vi "Configure Measure Mode.vi"(0 "VISA resource name":refnum<visa-resource-name>, 1 "MeasureMode (0=MyMeasure)":T1(ring), 5 "Show Table? (True)":bool=TRUE, 7 "Show Statistics? (True)":bool=TRUE, 9 "Show Histicons? (False)":bool, 11 "error in (no error)":errorcluster) -> (4 "VISA resource name out":refnum<visa-resource-name>, 15 "error out":errorcluster)   [LabVIEW 2018, in "LeCroy Wave Series.lvlib"]
doc: "Sets the Measure, Statistics and Histicon modes. (Note that histicons are not available on all series)\n\nIt is recommended to use this VI if you are configuring measurements programmatically rather than including them in a recalled panel setup file."
uses:
  LeCroy Wave Series.lvlib
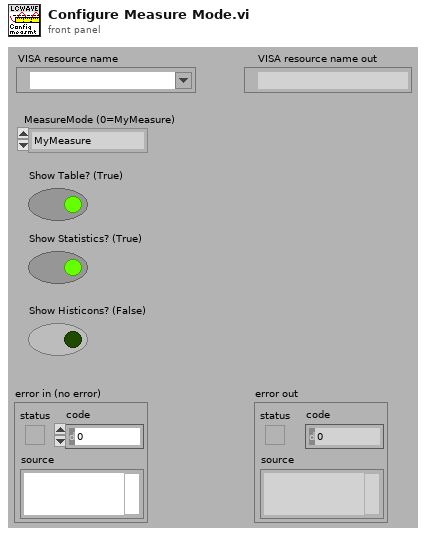
[diagram p1: front panel]
types:
  T1 = enum16{"MyMeasure", "Standard Vertical", "Standard Horizontal"}
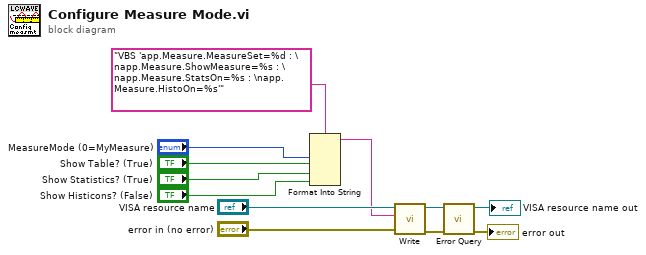
[diagram p0: block diagram]
diagram:
  n1 = Format Into String(format string="VBS 'app.Measure.MeasureSet=%d : \napp.Measure.ShowMeasure=%s : \napp.Measure.StatsOn=%s : \napp.Measure.HistoOn=%s'", "MeasureMode (0=MyMeasure)", "Show Table? (True)", "Show Statistics? (True)", "Show Histicons? (False)") -> (resulting string=w1:string)  [unwired: 2 in, 1 out]
  n2 = call "Write.vi"("error in (no error)"="error in (no error)", "Write Buffer"=w1, "VISA resource name"="VISA resource name") -> ("error out"=w8:errorcluster, "VISA resource name out"=w7:refnum<visa-resource-name>)  [unwired: 7 in]
  n3 = call "Error Query.vi"("error in (no error)"=w8, "VISA resource name"=w7) -> ("error out"=→"error out":errorcluster, "VISA resource name out"=→"VISA resource name out":refnum<visa-resource-name>)  [unwired: 6 in, 2 out]
